vi "Read.vi"(8 "error in (no error)":errorcluster, 9 "Timeout":i32=2000, 10 "NumOfBytes":i32=100, 11 "ClientBase in":refnum<class "ClientBase.lvclass">) -> (0 "error out":errorcluster, 2 "Data":string, 3 "ClientBase out":refnum<class "ClientBase.lvclass">)   [LabVIEW 2020, in "ClientBaseLib.lvlib" / "ClientBase.lvclass"]
uses:
  ClientBase.lvclass
  ClientBase.lvclass/ClientBase.ctl
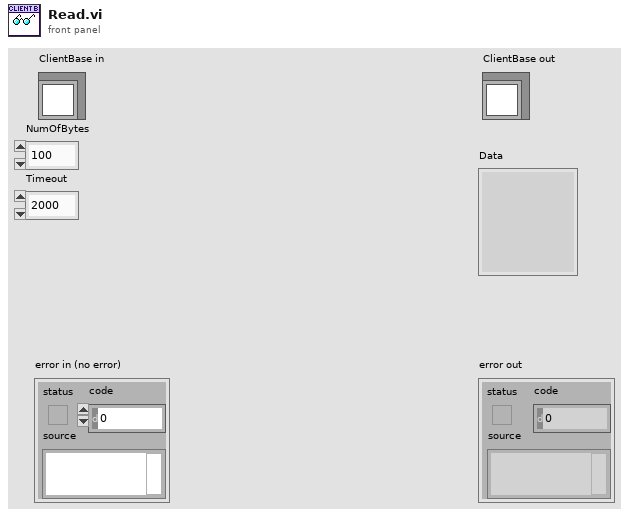
[diagram p1: front panel]
types:
  T1 = enum16{"Standard", "Buffered", "CRLF", "Immediate"}
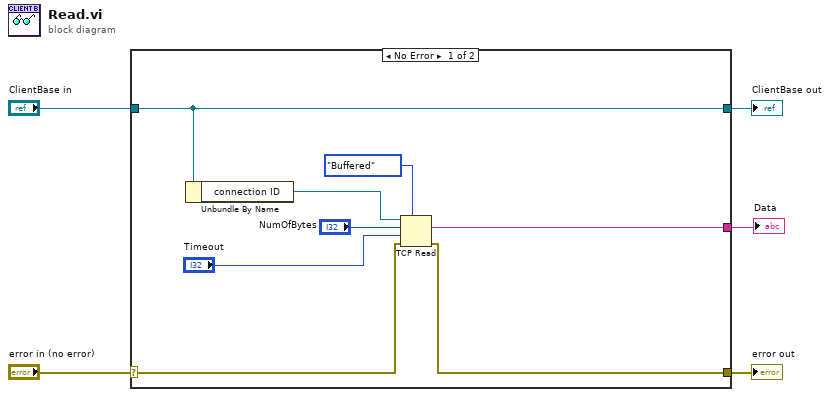
[diagram p0: block diagram]
diagram:
  n1 = case shown="No Error" "error in (no error)" {
    selector: "error in (no error)" -> [w9 w15]
    tunnel: [w8 w15] -> w4
    tunnel: [w13 w14] -> w2
    tunnel: "ClientBase in" -> [w13 w14]
    tunnel: [w6 _] -> w1
    frame No Error {
      n2 = Unbundle By Name(w13) -> ("connection ID"=w12:refnum<k5>)
      n3 = TCP Read(connection ID=w12, bytes to read="NumOfBytes", error in (no error)=w9, 7:T1."Buffered" ("mode (standard)"), 9:"Timeout") -> (data out=w6:string, error out=w8:errorcluster)  [unwired: 1 out]
    }
    frame Error {
    }
  }
  "error out" <- w4
  "ClientBase out" <- w2
  "Data" <- w1
